vi "Untitled 3 (SubVI).vi"() -> ()   [LabVIEW 2016]
panel:
  out "Boolean array":bool[][](array[boolean])
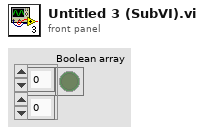
[diagram p1: front panel]
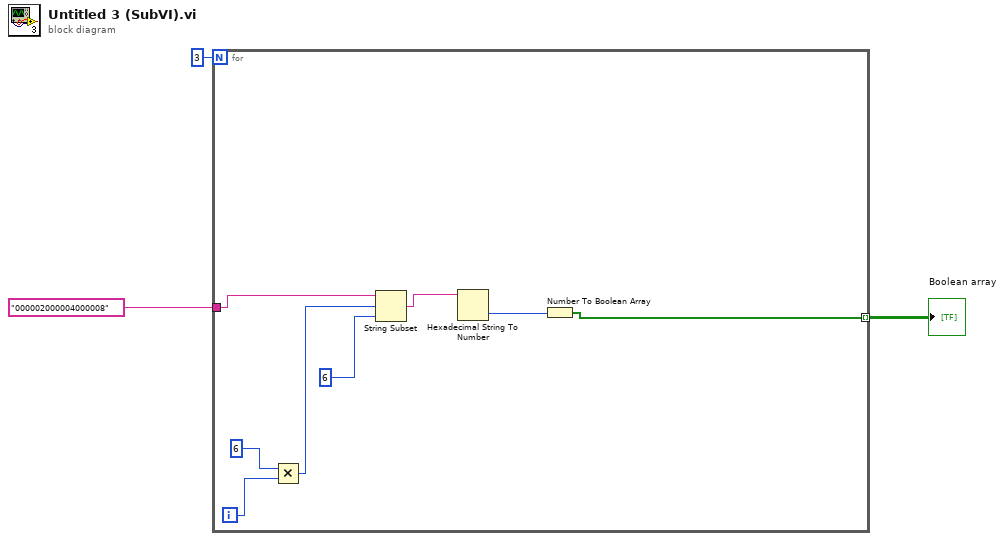
[diagram p0: block diagram]
diagram:
  n1 = for {
    N: 3 -> [_]
    tunnel: "000002000004000008" -> [w11]
    tunnel: [w4] -> w1 mode=indexing
    i -> [w9]
    n2 = Multiply(x=6, y=w9) -> (x*y=w7:i32)
    n3 = String Subset(string=w11, offset (0)=w7, length (rest)=6 ("length (rest)")) -> (substring=w6:string)
    n4 = Hexadecimal String To Number(string=w6) -> (number=w5:u32)  [unwired: 2 in, 1 out]
    n5 = Number To Boolean Array(number=w5) -> (Boolean array=w4:bool[])
  }
  "Boolean array" <- w1
